vi "Get Operations to Date.vi"(8 "error in (no error)":errorcluster caption="entrée d'erreur (pas d'erreur)", 10 "Date":timestamp, 11 "Operations en entrée":refnum<class "Operations.lvclass"> caption="DNL_LabVIEW Object in") -> (0 "error out":errorcluster caption="sortie d'erreur", 1 "Min Date":timestamp, 2 "Operations Found at Date":T1[](array[typedef]), 3 "Operations en sortie":refnum<class "Operations.lvclass"> caption="DNL_LabVIEW Object out")   [LabVIEW 2012, in "Operations.lvclass"]
uses:
  Operations.lvclass
  Operation/Operation Parameters.ctl
  Operation/Operation Type Enum.ctl
  controls/Currencies.ctl
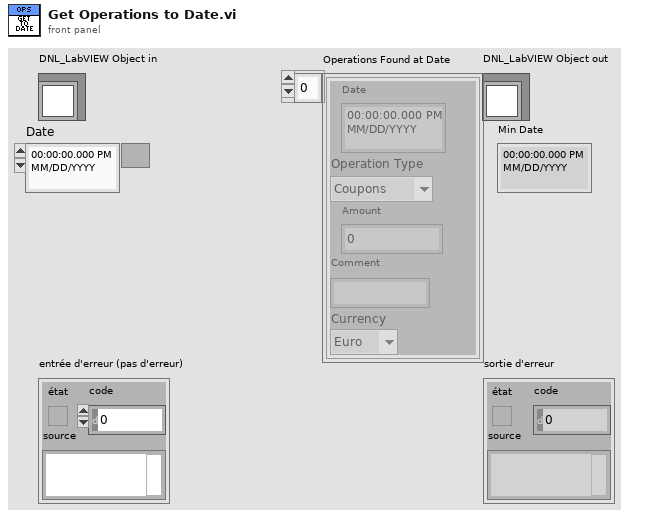
[diagram p1: front panel]
types:
  T1 = typedef "Operation Parameters.ctl" = cluster{"Date":timestamp, "Operation Type":T2, "Amount":dbl, "Comment":string, "Currency":T3}
  T2 = typedef "Operation Type Enum.ctl" = enum16{"Coupons", "Dépot", "Retrait", "Intérêts", "Taxe"}
  T3 = typedef "Currencies.ctl" = enum16{"Euro", "Dollar", "Yen", "RIM", "CHF"}
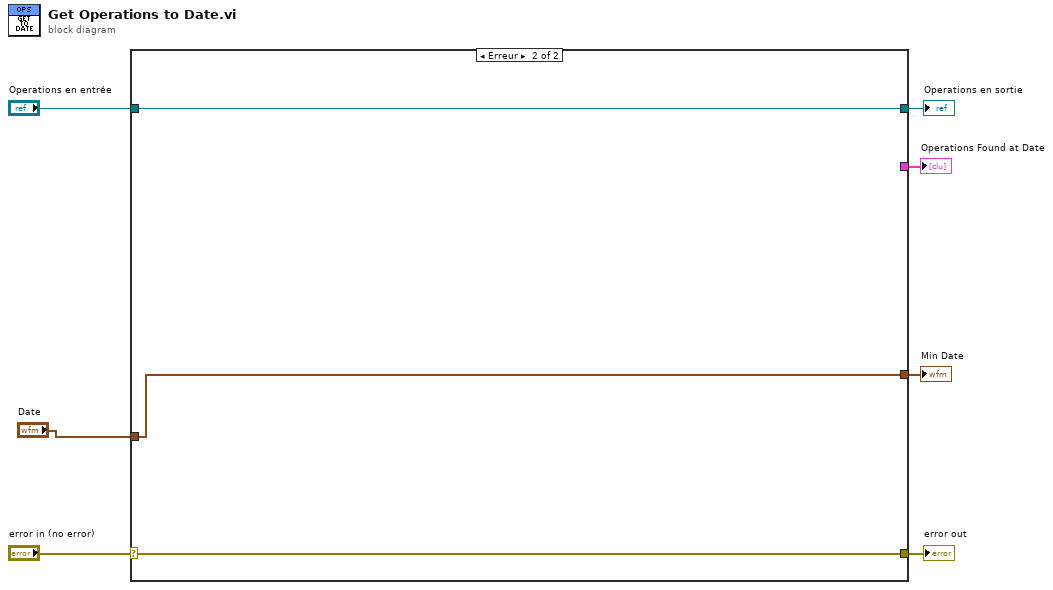
[diagram p0: block diagram]
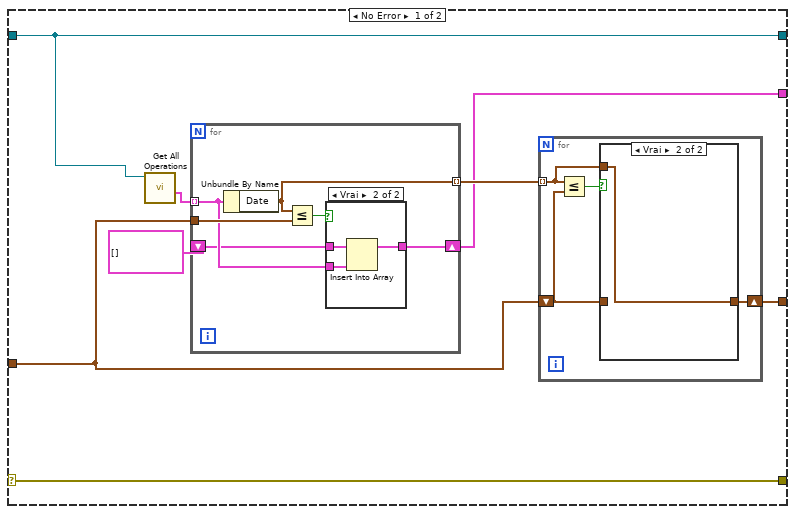
[diagram p2: hidden frame]
diagram:
  n1 = case shown="Erreur" "error in (no error)" {
    selector: "error in (no error)" -> [w15 w34]
    tunnel: [w15 w34] -> w6
    tunnel: [w10 w33] -> w4
    tunnel: "Operations en entrée" -> [w10 w33]
    tunnel: "Date" -> [w11 w32]
    tunnel: [w9 _] -> w2
    tunnel: [w8 w32] -> w1
    frame No Error {
      n2 = call "Get All Operations.vi"("Operations en entrée"=w10) -> ("Operations"=w14:T1[])  [unwired: 6 in, 4 out]
      n3 = for {
        tunnel: w14 -> [w25] mode=indexing
        tunnel: w11 -> [w27]
        shift-right: [w24] -> w9
        shift-left: T1[] [] -> [w23]
        tunnel: [w22] -> w12 mode=indexing
        n4 = Unbundle By Name(w25) -> ("Date"=w22:timestamp)
        n5 = Less Or Equal?(x=w22, y=w27) -> (x <= y?=w26:bool)
        n6 = case shown="Vrai" w26 {
          tunnel: w25 -> [_ w31]
          tunnel: [w28 w30] -> w24
          tunnel: w23 -> [w28 w29]
          frame False {
          }
          frame True {
            n7 = Insert Into Array(array=w29, new element=w31) -> (w30:T1[])  [unwired: 1 in]
          }
        }
      }
      n8 = for {
        tunnel: w12 -> [w18] mode=indexing
        shift-right: [w17] -> w8
        shift-left: w11 -> [w16]
        n9 = Less Or Equal?(x=w18, y=w16) -> (x <= y?=w19:bool)
        n10 = case shown="Vrai" w19 {
          tunnel: w18 -> [_ w21]
          tunnel: [w20 w21] -> w17
          tunnel: w16 -> [w20 _]
          frame False {
          }
          frame True {
          }
        }
      }
    }
    frame Error {
    }
  }
  "error out" <- w6
  "Operations en sortie" <- w4
  "Operations Found at Date" <- w2
  "Min Date" <- w1
